vi "write groundwater header csv file.vi"(6 "append to file? (new file:F)":bool=TRUE, 8 "error in (no error)":errorcluster, 9 "Groundwater Header":T1, 10 "Boolean":bool, 11 "Groundwater header file":path) -> (0 "error out":errorcluster)   [LabVIEW 2016]
uses:
  sdi_12/Groundwater header.ctl
  <vilib>/Utility/file.llb/Write Delimited Spreadsheet (string).vi
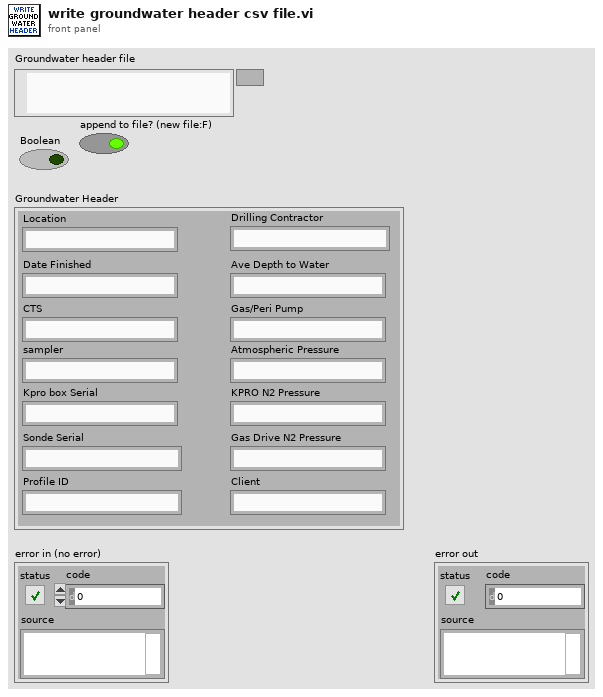
[diagram p1: front panel]
types:
  T1 = typedef "Groundwater header.ctl" = cluster{"Location":string, "Date Finished":string, "CTS":string, "sampler":string, "Kpro box Serial ":string, "Sonde Serial":string, "Drilling Contractor":string, "Ave Depth to Water":string, "Gas/Peri Pump":string, "Atmospheric Pressure":string, "KPRO N2 Pressure":string, "Gas Drive N2 Pressure":string, "Profile ID":string, "Client":string}
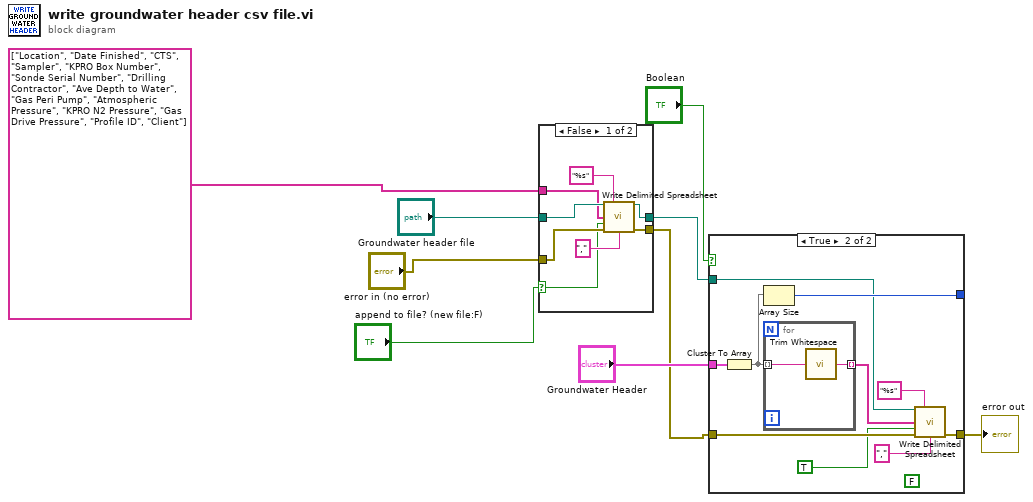
[diagram p0: block diagram]
diagram:
  n1 = case shown="False" "append to file? (new file:F)" {
    selector: "append to file? (new file:F)" -> [w12 _]
    tunnel: "Groundwater header file" -> [w16 w19]
    tunnel: [w11 w19] -> w4
    tunnel: [w15 w18] -> w2
    tunnel: "error in (no error)" -> [w14 w18]
    tunnel: string[] ["Location", "Date Finished", "CTS", "Sampler", "KPRO Box Number", "Sonde Serial Number", "Drilling Contractor", "Ave Depth to Water", "Gas Peri Pump", "Atmospheric Pressure", "KPRO N2 Pressure", "Gas Drive Pressure", "Profile ID", "Client"] -> [w10 _]
    frame False {
      n2 = call-poly <vilib>:"Write Delimited Spreadsheet.vi"("file path (dialog if empty)"=w16, "format (%s)"="%s" ("format (%.3f)"), "1D data"=w10, "append to file? (new file:F)"=w12, "error in (no error)"=w14, "delimiter (\\t)"="," ("delimiter (\\t)")) -> ("new file path (Not A Path if cancelled)"=w11:path, "error out"=w15:errorcluster)  [unwired: 8 in]
    }
    frame True {
    }
  }
  n3 = case shown="True" "Boolean" {
    tunnel: [w20 w28] -> w8
    tunnel: w2 -> [w20 w27]
    tunnel: [_ w24] -> _
    tunnel: "Groundwater Header" -> [_ w23]
    tunnel: w4 -> [_ w22]
    frame False {
    }
    frame True {
      (unwired) FALSE ("append to file? (new file:F)")
      n4 = Cluster To Array(cluster=w23) -> (array=w25:string[])
      n5 = Array Size(array=w25) -> (size(s)=w24:i32)
      n6 = for {
        tunnel: w25 -> [w32] mode=indexing
        tunnel: [w31] -> w26 mode=indexing
        n7 = call <vilib>:"Trim Whitespace.vi"("string"=w32) -> ("trimmed string"=w31:string)  [unwired: 1 in]
      }
      n8 = call-poly <vilib>:"Write Delimited Spreadsheet.vi"("file path (dialog if empty)"=w22, "format (%s)"="%s" ("format (%.3f)"), "1D data"=w26, "append to file? (new file:F)"=TRUE, "error in (no error)"=w27, "delimiter (\\t)"="," ("delimiter (\\t)")) -> ("error out"=w28:errorcluster)  [unwired: 8 in, 1 out]
    }
  }
  "error out" <- w8
